vi "Update RPC Method Template.vi"(8 "error in (no error)":errorcluster, 11 "Server Library (Library Item) in":refnum<vi>) -> (0 "error out":errorcluster, 3 "Server Library (Library Item) out":refnum<vi>)   [LabVIEW 2019, in "gRPC Template Creation Utility.lvlib"]
uses:
  gRPC Template Creation Utility.lvlib
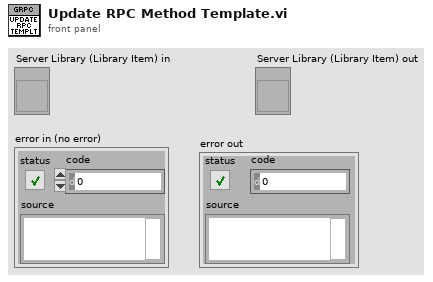
[diagram p1: front panel]
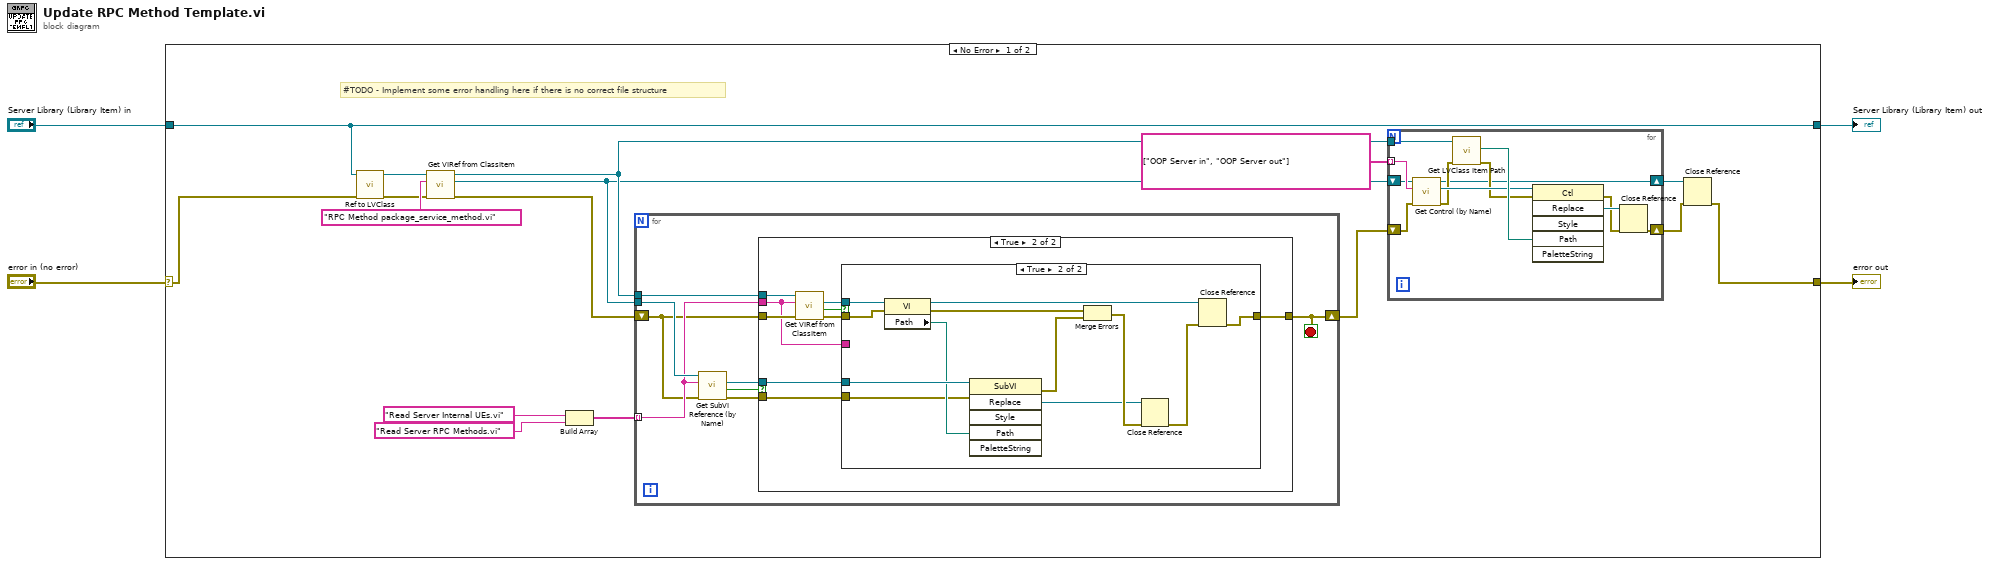
[diagram p0: block diagram]
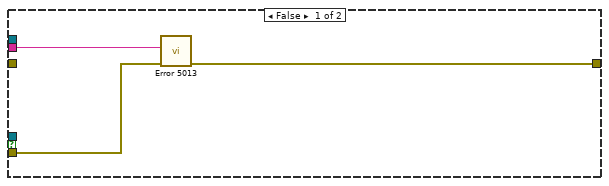
[diagram p2: hidden frame]
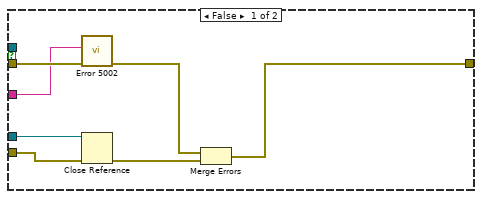
[diagram p3: hidden frame]
diagram:
  n1 = case shown="No Error" "error in (no error)" {
    selector: "error in (no error)" -> [w9 w73]
    tunnel: "Server Library (Library Item) in" -> [w7 w72]
    tunnel: [w10 w73] -> w3
    tunnel: [w7 w72] -> w1
    frame No Error {
      # "#TODO - Implement some error handling here if there is no correct file structure"
      n2 = call "Ref to LVClass.vi"("error in (no error)"=w9, "ProjectItem in"=w7) -> ("error out"=w8:errorcluster, "LVClassLibrary out"=w6:refnum<vi>)  [unwired: 8 in]
      n3 = call "Get VIRef from ClassItem.vi"("error in (no error)"=w8, "Item Name"="RPC Method package_service_method.vi", "LVClassLibrary in"=w6) -> ("error out"=w15:errorcluster, "VIref out"=w19:refnum<vi>, "LVClassLibrary out"=w20:refnum<vi>)  [unwired: 5 in, 1 out]
      n4 = Build Array("Read Server Internal UEs.vi" ("SubVI Name"), "Read Server RPC Methods.vi" ("SubVI Name")) -> (w18:string[])
      n5 = for {
        tunnel: w19 -> [w40]
        tunnel: w18 -> [w35] mode=indexing
        shift-right: [w37] -> w13
        shift-left: w15 -> [w33]
        tunnel: w20 -> [w34]
        stop <- w37 stop-if-true
        n6 = call "Get SubVI Reference (by Name).vi"("error in (no error)"=w33, "SubVI Name"=w35, "Owner VI in"=w40) -> ("error out"=w38:errorcluster, "Found ?"=w36:bool, "SubVI Refnum out"=w39:refnum<vi>)  [unwired: 5 in, 1 out]
        n7 = case shown="True" w36 {
          tunnel: w39 -> [_ w52]
          tunnel: w33 -> [_ w48]
          tunnel: w38 -> [w43 w51]
          tunnel: [w41 w50] -> w37
          tunnel: w34 -> [_ w49]
          tunnel: w35 -> [w42 w44]
          frame False {
            n8 = call "Error 5013.vi"("error in (no error)"=w43, "Element Name"=w42) -> ("error out"=w41:errorcluster)  [unwired: 9 in]
          }
          frame True {
            n9 = call "Get VIRef from ClassItem.vi"("error in (no error)"=w48, "Item Name"=w44, "LVClassLibrary in"=w49) -> ("error out"=w46:errorcluster, "Found ?"=w45:bool, "VIref out"=w47:refnum<vi>)  [unwired: 5 in, 1 out]
            n10 = case shown="True" w45 {
              tunnel: w52 -> [w59 w71]
              tunnel: w51 -> [w58 w69]
              tunnel: [w56 w63] -> w50
              tunnel: w47 -> [_ w61]
              tunnel: w46 -> [w55 w60]
              tunnel: w44 -> [w54 _]
              frame False {
                n11 = call "Error 5002.vi"("error in (no error)"=w55, "Method Name"=w54) -> ("error out"=w53:errorcluster)  [unwired: 9 in]
                n12 = Close Reference(reference=w59, error in (no error)=w58) -> (error out=w57:errorcluster)
                n13 = Merge Errors(w53, w57) -> (w56:errorcluster)
              }
              frame True {
                n14 = property class="VI"(reference=w61, error in=w60) -> (reference out=w64:refnum<vi>, error out=w67:errorcluster, "Path"=w70:path)
                n15 = invoke class="SubVI" method="Replace"(reference=w71, error in=w69, "Path"=w70) -> (error out=w68:errorcluster, "Replace"=w65:refnum<vi>)  [unwired: 3 in, 4 out]
                n16 = Merge Errors(w67, w68) -> (w66:errorcluster)
                n17 = Close Reference(reference=w65, error in (no error)=w66) -> (error out=w62:errorcluster)
                n18 = Close Reference(reference=w64, error in (no error)=w62) -> (error out=w63:errorcluster)
              }
            }
          }
        }
      }
      n19 = for {
        tunnel: w20 -> [w31]
        tunnel: string[] ["OOP Server in", "OOP Server out"] -> [w29] mode=indexing
        shift-right: [w21] -> w11
        shift-left: w19 -> [w28]
        shift-right: [w22] -> w12
        shift-left: w13 -> [w26]
        n20 = call "Get Control (by Name).vi"("error in (no error)"=w26, "Control Label"=w29, "Owner VI in"=w28) -> ("error out"=w27:errorcluster, "Control Refnum"=w30:refnum<vi>, "Owner VI out"=w21:refnum<vi>)  [unwired: 5 in, 1 out]
        n21 = call "Get LVClass Item Path.vi"("error in (no error)"=w27, "LVClassLibrary in"=w31) -> ("error out"=w25:errorcluster, "Path"=w32:path)  [unwired: 7 in, 1 out]
        n22 = invoke class="Ctl" method="Replace"(reference=w30, error in=w25, "Path"=w32) -> (error out=w23:errorcluster, "Replace"=w24:refnum<vi>)  [unwired: 3 in, 4 out]
        n23 = Close Reference(reference=w24, error in (no error)=w23) -> (error out=w22:errorcluster)
      }
      n24 = Close Reference(reference=w11, error in (no error)=w12) -> (error out=w10:errorcluster)
    }
    frame Error {
    }
  }
  "error out" <- w3
  "Server Library (Library Item) out" <- w1
